vi "Blit Scaled (Clusters).vi"(6 "Destination Rectangle":T1, 8 "error in":errorcluster, 9 "Destination Surface Pointer":u32 format="%.0x", 10 "Source Rectangle":T1, 11 "Source Surface Pointer":u32 format="%.0x") -> (0 "error out":errorcluster, 3 "Return":i32)   [LabVIEW 2014, in "LibSDL2.lvlib"]
uses:
  LibSDL2.lvlib
  Controls/Rectangle.ctl
  DLL/SDL2.dll
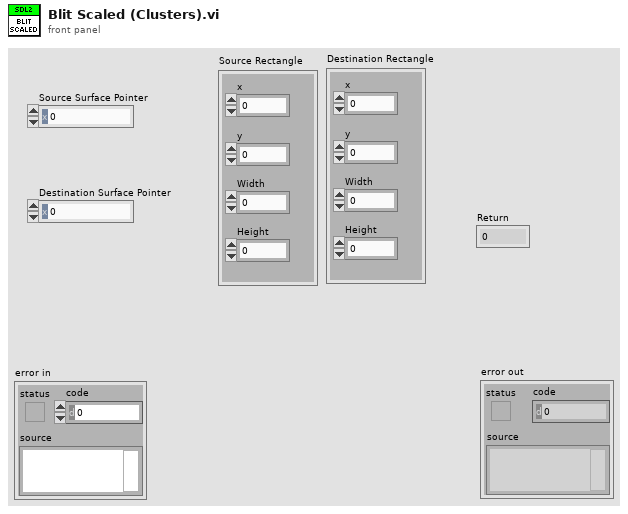
[diagram p1: front panel]
types:
  T1 = typedef "LibSDL2.lvlib/Rectangle.ctl" = cluster{"x":i32, "y":i32, "Width":i32, "Height":i32}
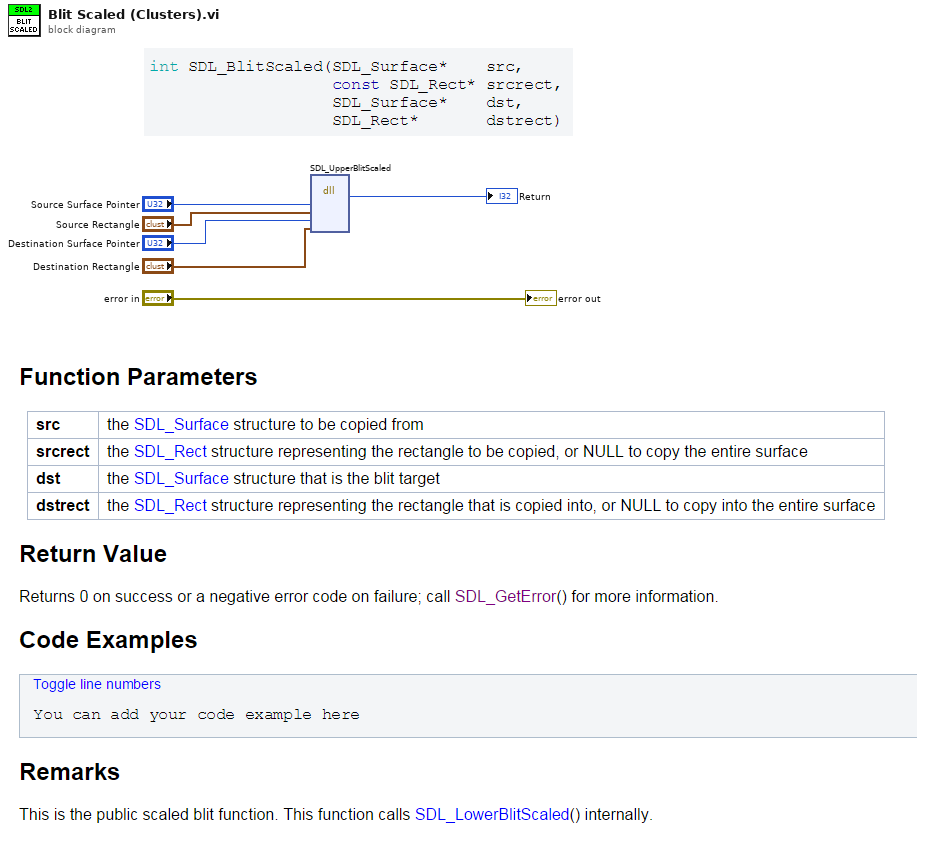
[diagram p0: block diagram]
diagram:
  n1 = dll-call lib="C:/dev/PGS/LabSDL2/Source/LibSDL2 Wrapper/DLL/SDL2.dll" fn="SDL_UpperBlitScaled"("src"="Source Surface Pointer", "srcrect"="Source Rectangle", "dst"="Destination Surface Pointer", "dstrect"="Destination Rectangle") -> ("return type"=→"Return":i32)  [unwired: 7 in, 2 out]
  "error out" <- "error in"
